vi "verlistaobjetosbase.vi"() -> (3 "lista_objetos":string[](array[string]))   [LabVIEW 2020]
doc: "Este VI devuelve la lista de objetos guardadas en la base de datos indicada en el archivo .udl contenida en la variable global de Path. Esta lista es mandada en el indicador de lista_objetos."
uses:
  Global_archivobasedatos.vi
  <vilib>/addons/database/Connection.llb/DB Tools Open Connec (Path).vi
  <vilib>/addons/database/Connection.llb/Conn Execute.vi
  <vilib>/addons/database/Recordset.llb/Rec Fetch Recordset Data (R).vi
  <vilib>/addons/database/Recordset.llb/Rec Destroy - Connection.vi
  <vilib>/addons/database/_DB Variant To Data/Database Variant To Data.xnode
  <vilib>/addons/database/NI_Database_API.lvlib
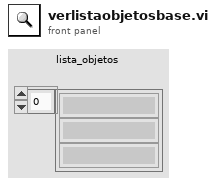
[diagram p1: front panel]
types:
  T1 = typedef "NI_Database_API.lvlib/Conn ObjectReference.ctl" = refnum<k1>
  T2 = typedef "NI_Database_API.lvlib/Rec ObjectReference.ctl" = refnum<k1>
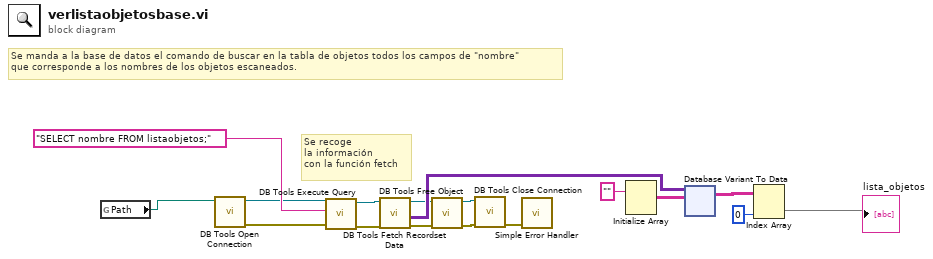
[diagram p0: block diagram]
diagram:
  # "Se recoge \nla información\ncon la función fetch"
  # "Se manda a la base de datos el comando de buscar en la tabla de objetos todos los campos de \"nombre\"\nque corresponde a los nombres de los objetos escaneados."
  n1 = global read "Global_archivobasedatos.vi" "Path"() -> (w9:path)
  n2 = call-poly <vilib>:"DB Tools Open Connection.vi"("connection information"=w9) -> ("error out"=w2:errorcluster, "connection reference"=w1:T1)  [unwired: 7 in]
  n3 = call-poly <vilib>:"DB Tools Execute Query.vi"("error in (no error)"=w2, "SQL query"="SELECT nombre FROM listaobjetos;", "connection reference"=w1) -> ("error out"=w4:errorcluster, "recordset reference"=w3:T2)  [unwired: 5 in]
  n4 = call-poly <vilib>:"DB Tools Fetch Recordset Data.vi"("error in (no error)"=w4, "recordset reference"=w3) -> ("error out"=w6:errorcluster, "recordset data"=w14:variant[][], "recordset reference out"=w5:T2)  [unwired: 3 in]
  n5 = call-poly <vilib>:"DB Tools Free Object.vi"("error in (no error)"=w6, "recordset reference"=w5) -> ("error out"=w13:errorcluster, "connection reference"=w11:T1)  [unwired: 8 in]
  n6 = call <vilib>:"DB Tools Close Connection.vi"("error in (no error)"=w13, "connection reference"=w11) -> ("error out"=w12:errorcluster)  [unwired: 5 in]
  n7 = call <vilib>:"Simple Error Handler.vi"("error in (no error)"=w12) -> ()  [unwired: 4 in, 5 out]
  n8 = Initialize Array("") -> (w8:string[][])  [unwired: 2 in]
  n9 = xnode "Database Variant To Data"("database variant"=w14, "type"=w8) -> ("data"=w15:string[][])  [unwired: 1 in, 1 out]
  n10 = Index Array(array=w15, index (col)=0 ("disabled index (col)")) -> (element=→"lista_objetos":string[])  [unwired: 1 in]
